vi "Configure Concurrent Measurements.vi"(8 "error in (no error)":errorcluster, 9 "Measurement Selection (3: Volts, Current)":u16(ring)=3 items=["Volts", "Current", "Resistance", "Volt, Current", "Volts, Resistance", "Current, Resistance", "All"], 10 "Enable Concurrent Measurements (F: Disable)":bool, 11 "VISA resource name":refnum<visa-resource-name>) -> (0 "error out":errorcluster, 3 "VISA resource name out":refnum<visa-resource-name>)   [LabVIEW 2019, in "Keithley 24XX.lvlib"]
doc: "Configures the instrument to use the selected measurements and only return these.\nConcurrent Measurements means that more than just Voltage or Current is measured at the same time.\nTo prevent data being sent that you don't need use the Configure Data Communication Format.vi"
uses:
  Keithley 24XX.lvlib
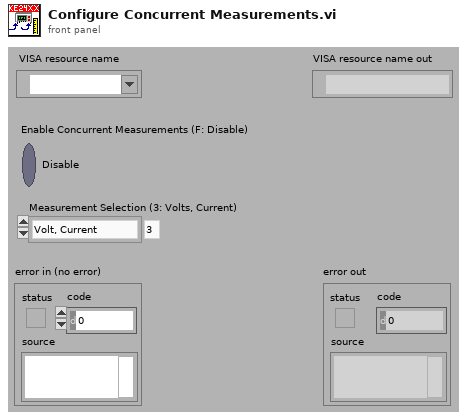
[diagram p1: front panel]
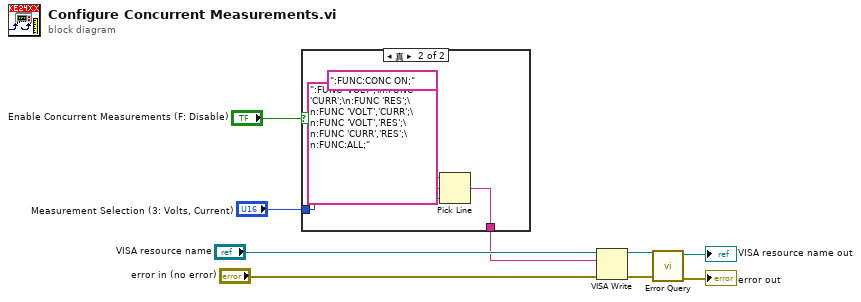
[diagram p0: block diagram]
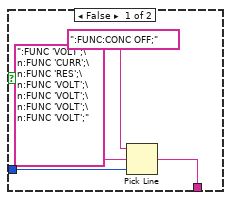
[diagram p2: hidden frame]
diagram:
  n1 = case shown="真" "Enable Concurrent Measurements (F: Disable)" {
    tunnel: [w13 w15] -> w3
    tunnel: "Measurement Selection (3: Volts, Current)" -> [w10 w14]
    frame False {
      n2 = Pick Line(string ("")=":FUNC:CONC OFF;", multi-line string=":FUNC 'VOLT';\n:FUNC 'CURR';\n:FUNC 'RES';\n:FUNC 'VOLT';\n:FUNC 'VOLT';\n:FUNC 'VOLT';\n:FUNC 'VOLT';", line index=w10) -> (output string=w13:string)
    }
    frame True {
      n3 = Pick Line(string ("")=":FUNC:CONC ON;", multi-line string=":FUNC 'VOLT';\n:FUNC 'CURR';\n:FUNC 'RES';\n:FUNC 'VOLT','CURR';\n:FUNC 'VOLT','RES';\n:FUNC 'CURR','RES';\n:FUNC:ALL;", line index=w14) -> (output string=w15:string)
    }
  }
  n4 = VISA Write(VISA resource name="VISA resource name", write buffer=w3, error in (no error)="error in (no error)") -> (VISA resource name out=w6:refnum<visa-resource-name>, error out=w7:errorcluster)  [unwired: 1 out]
  n5 = call "Error Query.vi"("error in (no error)"=w7, "VISA resource name"=w6) -> ("error out"=→"error out":errorcluster, "VISA resource name out"=→"VISA resource name out":refnum<visa-resource-name>)  [unwired: 6 in, 2 out]
